vi "TETRIX Motor(s) Move_HT_myRIO.vi"(0 "Motor 2 Power (-100 to 100)\n0 = Stop/Brake\n-128 = Stop/Coast":i8(slide) scale=-100.0..100.0, 1 "Motor 1 Power (-100 to 100)\n0 = Stop/Brake\n-128 = Stop/Coast":i8(slide) scale=-100.0..100.0, 2 "Control Mode":string(combo)="Power Only", 4 "Motor 2 Reverse? : T or F":bool, 5 "Motor 1 Reverse? : T or F":bool, 6 "Encoder 2 Target: 360 = 1 motor shaft revolution":i32, 7 "Encoder 1 Target: 360 = 1 motor shaft revolution":i32, 8 "Controller Daisy Chain Position: 1 - 4":u8=1, 9 "error in (no error)":errorcluster) -> (3 "error out":errorcluster)   [LabVIEW 2014]
uses:
  <vilib>/myRIO/Instrument Drivers/Onboard IO/I2C/vis/Configure.vi
  <vilib>/myRIO/Instrument Drivers/Onboard IO/I2C/vis/Write.vi
  <vilib>/myRIO/Instrument Drivers/Onboard IO/I2C/vis/Smart Open.vi
  <vilib>/Utility/error.llb/Error Cluster From Error Code.vi
  <vilib>/myRIO/Common/Instrument Driver Framework/myRIO v1.0/I2C/vis/myRIO v1.0 Configure I2C.vi
  <vilib>/myRIO/Common/Instrument Driver Framework/myRIO v1.0/I2C/vis/myRIO v1.0 Write I2C.vi
panel:
  # "TETRIX_HT Move Motor(s) VI"
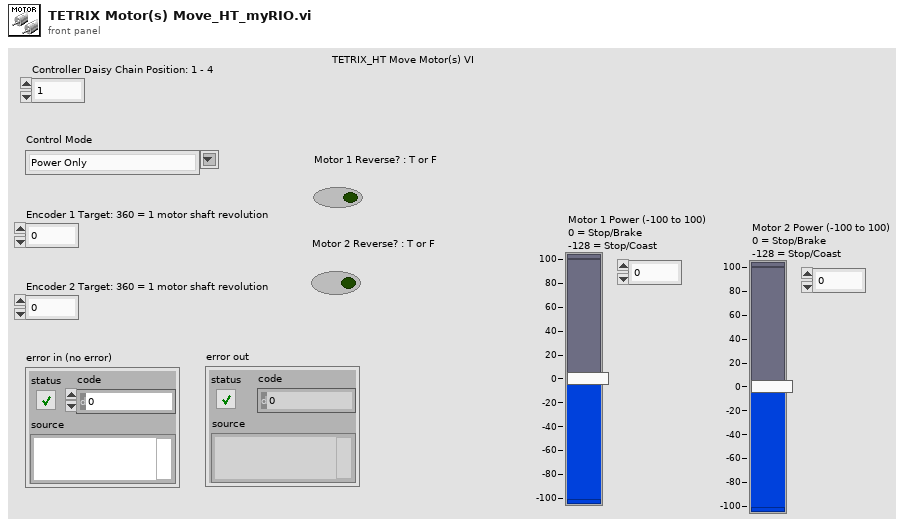
[diagram p1: front panel]
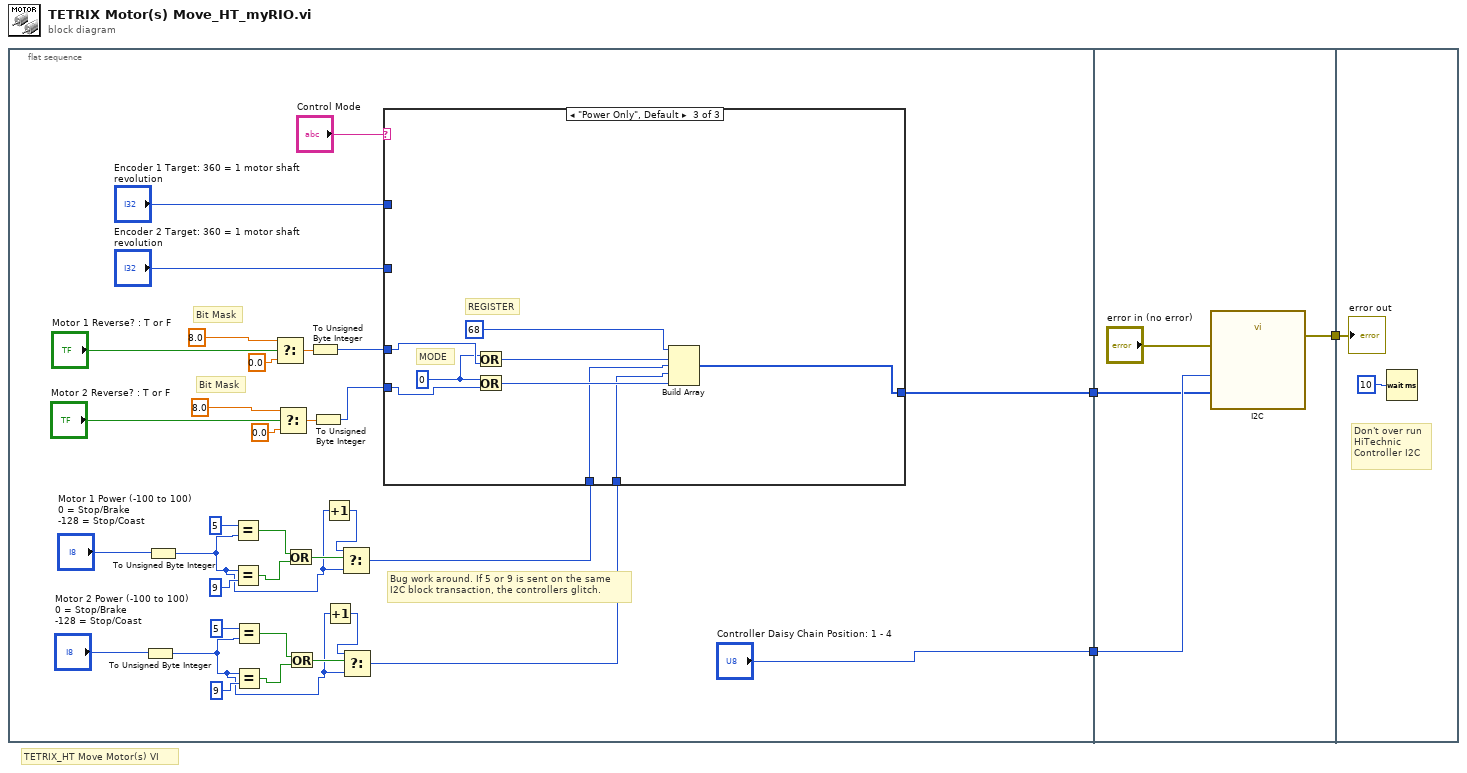
[diagram p0: block diagram]
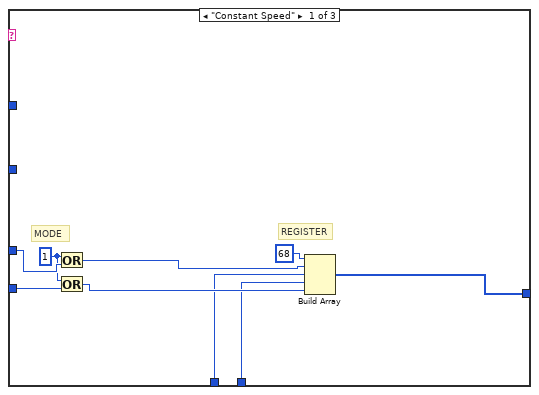
[diagram p2: hidden frame]
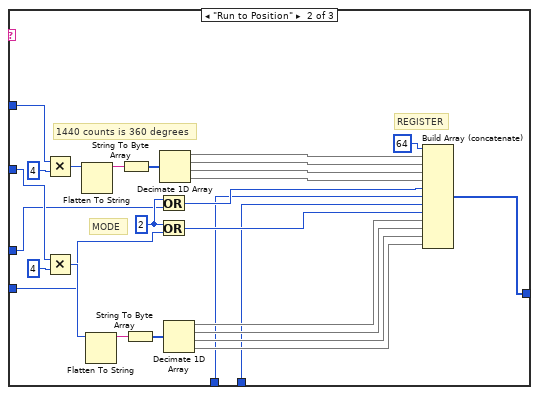
[diagram p3: hidden frame]
diagram:
  # "TETRIX_HT Move Motor(s) VI"
  n1 = flat-sequence {
    tunnel: ["Controller Daisy Chain Position: 1 - 4"] -> w3
    tunnel: [w22] -> w2
    tunnel: [w85] -> w1
    tunnel: w3 -> [w83]
    tunnel: w2 -> [w82]
    tunnel: w1 -> [w86]
    frame #0 {
      # "Bug work around. If 5 or 9 is sent on the same\nI2C block transaction, the controllers glitch."
      # "Bit Mask"
      # "Bit Mask"
      n2 = To Unsigned Byte Integer(number="Motor 2 Power (-100 to 100)\n0 = Stop/Brake\n-128 = Stop/Coast") -> (unsigned 8bit integer=w6:u8)
      n3 = To Unsigned Byte Integer(number="Motor 1 Power (-100 to 100)\n0 = Stop/Brake\n-128 = Stop/Coast") -> (unsigned 8bit integer=w13:u8)
      n4 = Equal?(x=u8 5, y=w13) -> (x = y?=w17:bool)
      n5 = Equal?(x=w13, y=u8 9) -> (x = y?=w16:bool)
      n6 = Equal?(x=u8 5, y=w6) -> (x = y?=w10:bool)
      n7 = Equal?(x=w6, y=u8 9) -> (x = y?=w9:bool)
      n8 = Select(t=8.0, s="Motor 1 Reverse? : T or F", f=0.0) -> (s? t:f=w33:dbl)
      n9 = Select(t=8.0, s="Motor 2 Reverse? : T or F", f=0.0) -> (s? t:f=w28:dbl)
      n10 = Or(x=w17, y=w16) -> (x .or. y?=w15:bool)
      n11 = Or(x=w10, y=w9) -> (x .or. y?=w8:bool)
      n12 = To Unsigned Byte Integer(number=w33) -> (unsigned 8bit integer=w25:u8)
      n13 = To Unsigned Byte Integer(number=w28) -> (unsigned 8bit integer=w24:u8)
      n14 = Increment(x=w13) -> (x+1=w14:u8)
      n15 = Increment(x=w6) -> (x+1=w7:u8)
      n16 = Select(t=w14, s=w15, f=w13) -> (s? t:f=w5:u8)
      n17 = Select(t=w7, s=w8, f=w6) -> (s? t:f=w4:u8)
      n18 = case shown="\"Power Only\", Default" "Control Mode" {
        tunnel: "Encoder 1 Target: 360 = 1 motor shaft revolution" -> [_ w68 _]
        tunnel: "Encoder 2 Target: 360 = 1 motor shaft revolution" -> [_ w63 _]
        tunnel: w25 -> [w44 w52 w80]
        tunnel: w24 -> [w45 w51 w79]
        tunnel: [w41 w50 w77] -> w22
        tunnel: w5 -> [w38 w47 w74]
        tunnel: w4 -> [w37 w46 w73]
        frame "Constant Speed" {
          w43 = u8 1
          # "REGISTER"
          # "MODE"
          n19 = Or(x=w43, y=w44) -> (x .or. y?=w40:u8)
          n20 = Or(x=w43, y=w45) -> (x .or. y?=w39:u8)
          n21 = Build Array(u8 68 ("element"), w40, w38, w37, w39) -> (w41:u8[])
        }
        frame "Run to Position" {
          w53 = u8 2
          # "1440 counts is 360 degrees"
          # "REGISTER"
          # "MODE"
          n22 = Multiply(x=w68, y=4) -> (x*y=w72:i32)
          n23 = Multiply(x=w63, y=4) -> (x*y=w66:i32)
          n24 = Flatten To String(anything=w72) -> (data string=w69:string)  [unwired: 3 in, 2 out]
          n25 = Flatten To String(anything=w66) -> (data string=w64:string)  [unwired: 3 in, 2 out]
          n26 = String To Byte Array(string=w69) -> (unsigned byte array=w70:u8[])
          n27 = String To Byte Array(string=w64) -> (unsigned byte array=w65:u8[])
          n28 = Or(x=w53, y=w52) -> (x .or. y?=w49:u8)
          n29 = Or(x=w53, y=w51) -> (x .or. y?=w48:u8)
          n30 = Decimate 1D Array(w70) -> (w61:u8[], w60:u8[], w59:u8[], w58:u8[])
          n31 = Decimate 1D Array(w65) -> (w54:u8[], w55:u8[], w56:u8[], w57:u8[])
          n32 = Build Array (concatenate)(u8 64 ("element"), w61, w60, w59, w58, w49, w47, w46, w48, w54, w55, w56, w57) -> (w50:u8[])
        }
        frame "Power Only", Default {
          w78 = u8 0
          # "MODE"
          # "REGISTER"
          n33 = Or(x=w78, y=w80) -> (x .or. y?=w76:u8)
          n34 = Or(x=w78, y=w79) -> (x .or. y?=w75:u8)
          n35 = Build Array(u8 68 ("element"), w76, w74, w73, w75) -> (w77:u8[])
        }
      }
    }
    frame #1 {
      n36 = call "I2C"("Slave Address (7-bit)"=w83, "Bytes to Write"=w82, "error in (no error)"="error in (no error)") -> ("error out"=w85:errorcluster)  [unwired: 24 in]
    }
    frame #2 {
      # "Don't over run\nHiTechnic\nController I2C"
      n37 = Wait (ms)(milliseconds to wait=u32 10) -> ()  [unwired: 1 out]
      "error out" <- w86
    }
  }
